vi "KMRmOS6DeltaRCMotorControl.vi"(8 "error in (no error)":errorcluster, 9 "Theta3":dbl, 10 "Theta2":dbl, 11 "Theta1":dbl) -> (0 "error out":errorcluster)   [LabVIEW 2019]
uses:
  KNRm_ReMi_OS6_436Motor.lvlibp/KNRm_ReMi_Toolkit/IO/LowLevel/IO_Channel_RC.ctl
  math/Global 1.vi
  KNRm_ReMi_OS6_436Motor.lvlibp
panel:
  out "coerced(x)":dbl
  out "x/y":dbl
  out "x+y":dbl
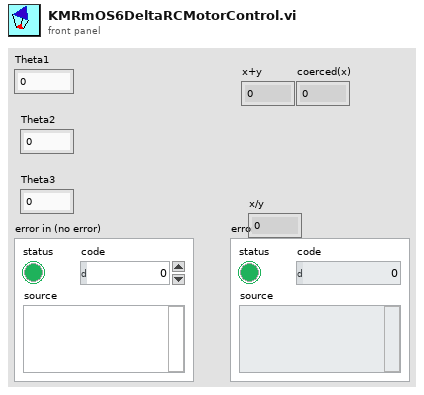
[diagram p1: front panel]
types:
  T1 = cluster{"等比調整到角度正確":cluster{"S1":dbl, "S2":dbl, "S3":dbl, "S4":dbl, "S5":dbl}, "補償角度到0度是水平":cluster{"S1":dbl, "S2":dbl, "S3":dbl, "S4":dbl, "S5":dbl}}
  T2 = typedef "KNRm_ReMi_OS6_436Motor.lvlibp/IO_Channel_RC.ctl" = enum16{"RC1", "RC2", "S1(EXTIOB)", "S2(EXTIOB)", "S3(EXTIOB)", "S4(EXTIOB)", "S5(EXTIOB)", "S6(EXTIOB)"}
  T3 = cluster{"S1":dbl, "S2":dbl, "S3":dbl, "S4":dbl, "S5":dbl}
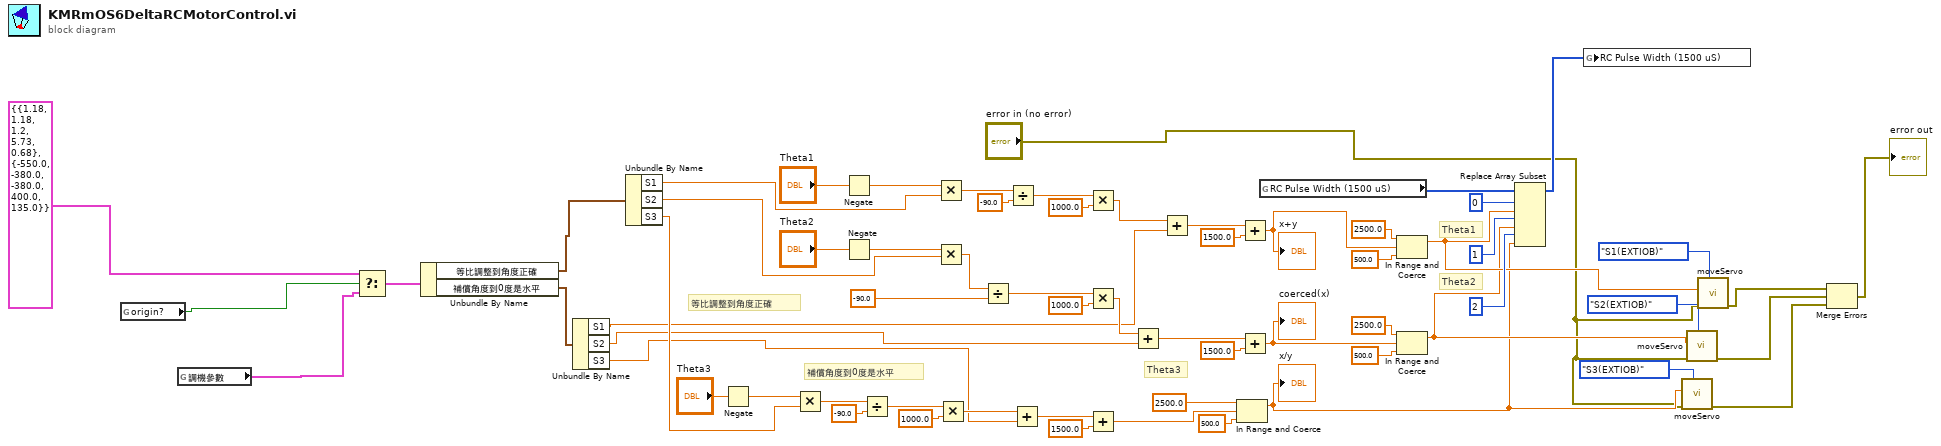
[diagram p0: block diagram]
diagram:
  # "補償角度到0度是水平"
  # "等比調整到角度正確"
  # "Theta2"
  # "Theta3"
  # "Theta1"
  n1 = global read "Global 1.vi" "origin?"() -> (w21:bool)
  n2 = global read "Global 1.vi" "調機參數"() -> (w22:T1)
  n3 = Select(t=T1 {"等比調整到角度正確"={"S1"=1.18, "S2"=1.18, "S3"=1.2, "S4"=5.73, "S5"=0.68}, "補償角度到0度是水平"={"S1"=-550.0, "S2"=-380.0, "S3"=-380.0, "S4"=400.0, "S5"=135.0}} ("調機參數"), s=w21, f=w22) -> (s? t:f=w23:T1)
  n4 = Unbundle By Name(w23) -> ("等比調整到角度正確"=w9:T3, "補償角度到0度是水平"=w8:T3)
  n5 = Unbundle By Name(w8) -> ("S1"=w4:dbl, "S2"=w3:dbl, "S3"=w2:dbl)
  n6 = Unbundle By Name(w9) -> ("S1"=w7:dbl, "S2"=w6:dbl, "S3"=w5:dbl)
  n7 = Negate(x="Theta3") -> (-x=w38:dbl)
  n8 = Multiply(x=w38, y=w5) -> (x*y=w36:dbl)
  n9 = Negate(x="Theta1") -> (-x=w39:dbl)
  n10 = Negate(x="Theta2") -> (-x=w40:dbl)
  n11 = Divide(x=w36, y=-90.0) -> (x/y=w61:dbl)
  n12 = Multiply(x=w39, y=w7) -> (x*y=w37:dbl)
  n13 = Multiply(x=w40, y=w6) -> (x*y=w35:dbl)
  n14 = Multiply(x=w61, y=1000.0) -> (x*y=w30:dbl)
  n15 = Divide(x=w35, y=-90.0) -> (x/y=w53:dbl)
  n16 = Divide(x=w37, y=-90.0) -> (x/y=w57:dbl)
  n17 = Add(x=w30, y=w2) -> (x+y=w29:dbl)
  n18 = Multiply(x=w57, y=1000.0) -> (x*y=w32:dbl)
  n19 = Multiply(x=w53, y=1000.0) -> (x*y=w34:dbl)
  n20 = Add(x=w29, y=1500.0) -> (x+y=w46:dbl)
  n21 = Add(x=w34, y=w3) -> (x+y=w33:dbl)
  n22 = Add(x=w32, y=w4) -> (x+y=w31:dbl)
  n23 = In Range and Coerce(upper limit=2500.0, x=w46, lower limit=500.0) -> (coerced(x)=w11:dbl)  [unwired: 1 out]
  "x/y" <- w11
  n24 = Add(x=w31, y=1500.0) -> (x+y=w45:dbl)
  "x+y" <- w45
  n25 = Add(x=w33, y=1500.0) -> (x+y=w44:dbl)
  "coerced(x)" <- w44
  n26 = global read "Global 1.vi" "RC Pulse Width (1500 uS)"() -> (w28:u16[])
  n27 = In Range and Coerce(upper limit=2500.0, x=w45, lower limit=500.0) -> (coerced(x)=w13:dbl)  [unwired: 1 out]
  n28 = In Range and Coerce(upper limit=2500.0, x=w44, lower limit=500.0) -> (coerced(x)=w12:dbl)  [unwired: 1 out]
  n29 = Replace Array Subset(array=w28, new element #1=w13, index #1=0 ("index"), new element #2=w12, index #2=1 ("index"), new element #3=w11, index #3=2 ("index")) -> (w26:u16[])
  n30 = global write "Global 1.vi" "RC Pulse Width (1500 uS)"(w26) -> ()
  n31 = call "moveServo.vi"("Channel"=IO_Channel_RC."S3(EXTIOB)", "error in (no error)"="error in (no error)", "Servo Position (us)"=w11) -> ("error out"=w15:errorcluster)  [unwired: 8 in]
  n32 = call "moveServo.vi"("Channel"=IO_Channel_RC."S2(EXTIOB)", "error in (no error)"="error in (no error)", "Servo Position (us)"=w12) -> ("error out"=w16:errorcluster)  [unwired: 8 in]
  n33 = call "moveServo.vi"("Channel"=IO_Channel_RC."S1(EXTIOB)", "error in (no error)"="error in (no error)", "Servo Position (us)"=w13) -> ("error out"=w17:errorcluster)  [unwired: 8 in]
  n34 = Merge Errors(w17, w16, w15) -> (→"error out":errorcluster)
